vi "Add Employees Salary Info to Employee Salary Table.vi"(8 "error in (no error)":errorcluster caption="错误输入（无错误）", 10 "Employees Salary Info":T1[](array[typedef]), 11 "Employee 输入":refnum<class "Employee.lvclass"> caption="DNL_LabVIEW Object in") -> (0 "error out":errorcluster caption="错误输出", 3 "Employee 输出":refnum<class "Employee.lvclass"> caption="DNL_LabVIEW Object out")   [LabVIEW 2012, in "Employee.lvclass"]
uses:
  Employee.lvclass
  Custom Def/Salary Info.ctl
  Employee.lvclass/Employee.ctl
  Data Table/DataTable.lvclass
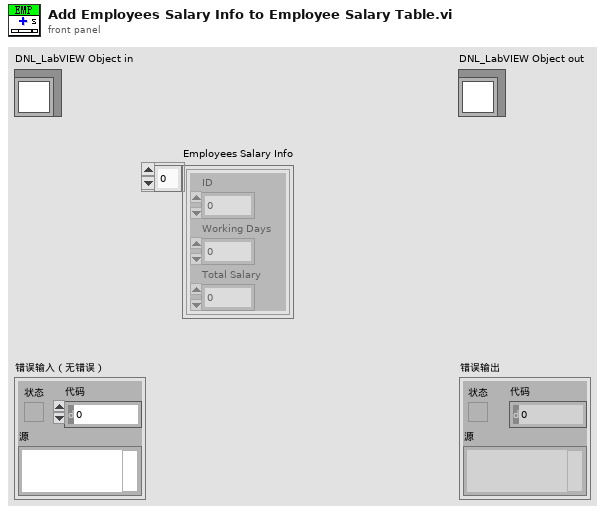
[diagram p1: front panel]
types:
  T1 = typedef "Salary Info.ctl" = cluster{"ID":u16, "Working Days":dbl, "Total Salary":dbl}
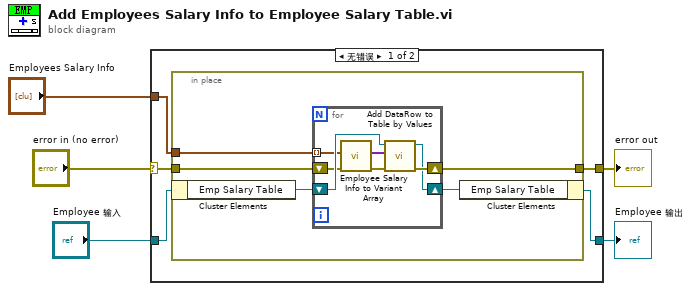
[diagram p0: block diagram]
diagram:
  n1 = case shown="无错误" "error in (no error)" {
    selector: "error in (no error)" -> [w8 w24]
    tunnel: [w7 w24] -> w4
    tunnel: [w6 w23] -> w2
    tunnel: "Employee 输入" -> [w10 w23]
    tunnel: "Employees Salary Info" -> [w9 _]
    frame No Error {
      n2 = in-place {
        in-place-border: w9 -> [w15]
        in-place-border: w8 -> [w12]
        in-place-border: [w11] -> w7
        n3 = in-place-cluster #1(w10) -> ("Emp Salary Table"=w14:refnum<class "DataTable.lvclass">)
        n4 = for {
          tunnel: w15 -> [w19] mode=indexing
          shift-right: [w20] -> w13
          shift-left: w14 -> [w22]
          shift-right: [w21] -> w11
          shift-left: w12 -> [w17]
          n5 = call "Employee Salary Info to Variant Array.vi"("error in (no error)"=w17, "Salary Info"=w19) -> ("error out"=w16:errorcluster, "Salary Variant Array"=w18:variant[])  [unwired: 7 in, 1 out]
          n6 = call "Add DataRow to Table by Values.vi"("error in (no error)"=w16, "values"=w18, "DataTable 输入"=w22) -> ("error out"=w21:errorcluster, "DataTable 输出"=w20:refnum<class "DataTable.lvclass">)  [unwired: 7 in]
        }
        n7 = in-place-cluster #1("Emp Salary Table"=w13) -> (w6:refnum<class "Employee.lvclass">)
      }
    }
    frame Error {
    }
  }
  "error out" <- w4
  "Employee 输出" <- w2
